vi "Set Node State.vi"(8 "Error In":errorcluster, 10 "CANopen Message":refnum<class "CANopen Response Message.lvclass">, 11 "reference in":refnum<class "Network Mangement.lvclass">) -> (0 "Error Out":errorcluster, 2 "New Node/State?":bool, 3 "reference out":refnum<class "Network Mangement.lvclass">)   [LabVIEW 2024, in "CANopen Master.lvlib" / "Network Mangement.lvclass"]
uses:
  Network Mangement.lvclass
  CANopen Response/CANopen Response Message.lvclass
  D:/git/CANopen-XNET/CANopen Message/CANopen Message.lvclass
  CANopen Message/CANopen Message.lvclass/CANopen Message.ctl
  Network Mangement.lvclass/Network Mangement.ctl
  CANopen Message/CANopen Message.lvclass
  D:/git/CANopen-XNET/CANopen Response/CANopen Response Message.lvclass
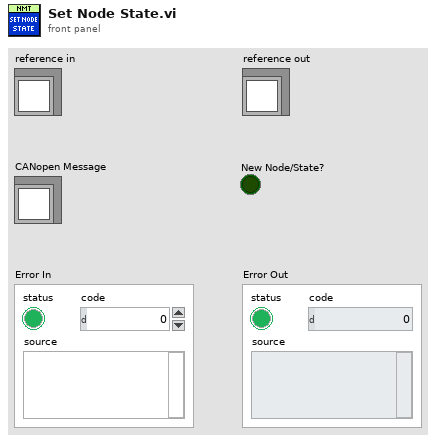
[diagram p1: front panel]
types:
  T1 = typedef "CANopen Master.lvlib/CANopen Response Message.lvclass/Server Command Specifier.ctl" = enum8{"Upload Segment Response", "Download Segment Response", "Initiate Upload Response", "Initiate Download Response", "Heartbeat", "Block Download"}
  T2 = typedef "CANopen Master.lvlib/Network Mangement.lvclass/ObjectAttributes.ctl" = cluster{"Nodes":map{u8, u8}}
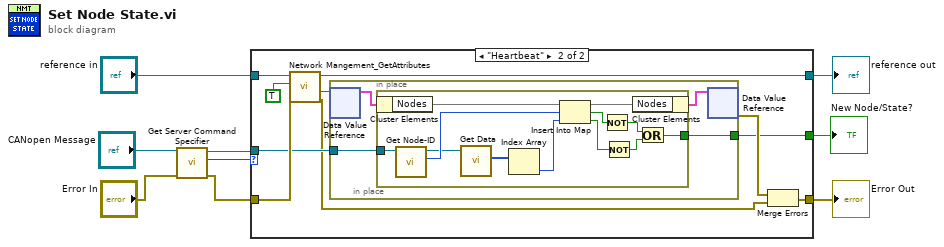
[diagram p0: block diagram]
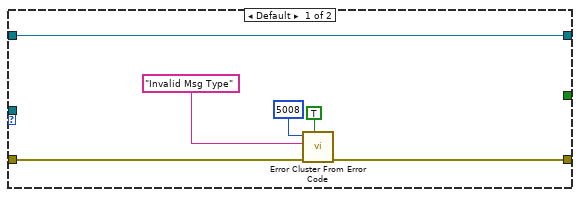
[diagram p2: hidden frame]
diagram:
  n1 = call-dynamic "Get Server Command Specifier.vi"("error in"="Error In", "CANopen Response in"="CANopen Message") -> ("error out"=w3:errorcluster, "Server Command Specifier"=w2:T1, "CANopen Response out"=w5:refnum<class "CANopen Response Message.lvclass">)  [unwired: 7 in]
  n2 = case shown="\"Heartbeat\"" w2 {
    tunnel: w3 -> [w15 w25]
    tunnel: [w13 w24] -> w9
    tunnel: "reference in" -> [w14 w23]
    tunnel: [w14 w22] -> w7
    tunnel: w5 -> [_ w18]
    tunnel: [_ w17] -> w1
    frame Default {
      n3 = call <vilib>:"Error Cluster From Error Code.vi"("show call chain? (False)"=TRUE, "error in (no error)"=w15, "error message (\"\")"="Invalid Msg Type" ("error message (\"\")"), "error code (0)"=5008) -> ("error out"=w13:errorcluster)  [unwired: 5 in]
    }
    frame "Heartbeat" {
      n4 = call "Network Mangement_GetAttributes.vi"("Error In"=w25, "OnlyGetDvrReference(False)"=TRUE, "reference in"=w23) -> ("Error Out"=w16:errorcluster, "DataRef"=w20:refnum<data-value>, "reference out"=w22:refnum<class "Network Mangement.lvclass">)  [unwired: 5 in, 1 out]
      n5 = in-place {
        in-place-border: w18 -> [w28]
        in-place-border: [w26] -> w17
        n6 = in-place-dvr #1(w20) -> (w29:T2)  [unwired: 1 out]
        n7 = in-place {
          in-place-border: w28 -> [w39]
          in-place-border: [w32] -> w26
          n8 = in-place-cluster #2(w29) -> ("Nodes"=w41:map{u8, u8})
          n9 = call "Get Node-ID.vi"("CANopen Message in"=w39) -> ("Node-ID"=w38:u8, "CANopen Message out"=w37:refnum<class "CANopen Response Message.lvclass">)  [unwired: 9 in]
          n10 = call "Get Data.vi"("CANopen Message in"=w37) -> ("Data"=w36:u8[])  [unwired: 9 in, 1 out]
          n11 = Index Array(array=w36) -> (element=w34:u8)  [unwired: 1 in]
          n12 = Insert Into Map(map in=w41, key=w38, value=w34) -> (map out=w40:map{u8, u8}, key already included?=w35:bool, value unchanged?=w30:bool)
          n13 = Not(x=w35) -> (.not. x?=w33:bool)
          n14 = Not(x=w30) -> (.not. x?=w31:bool)
          n15 = in-place-cluster #2("Nodes"=w40) -> (w27:T2)
          n16 = Or(x=w33, y=w31) -> (x .or. y?=w32:bool)
        }
        n17 = in-place-dvr #1(w27) -> (w19:errorcluster)  [unwired: 1 out]
      }
      n18 = Merge Errors(w19, w16) -> (w24:errorcluster)
    }
  }
  "Error Out" <- w9
  "reference out" <- w7
  "New Node/State?" <- w1
